vi "setROI.vi"(8 "error in (no error)":errorcluster, 10 "Coordinates":i32[](array[numeric]), 11 "ImageStreamViewer in":refnum<class "ImageStreamViewer.lvclass">) -> (0 "error out":errorcluster, 3 "ImageStreamViewer out":refnum<class "ImageStreamViewer.lvclass">)   [LabVIEW 2009, in "Views.lvlib" / "Camera.lvlib" / "ImageStreamViewer.lvclass"]
uses:
  ImageStreamViewer.lvclass
  ImageStreamViewer.lvclass/ImageStreamViewer.ctl
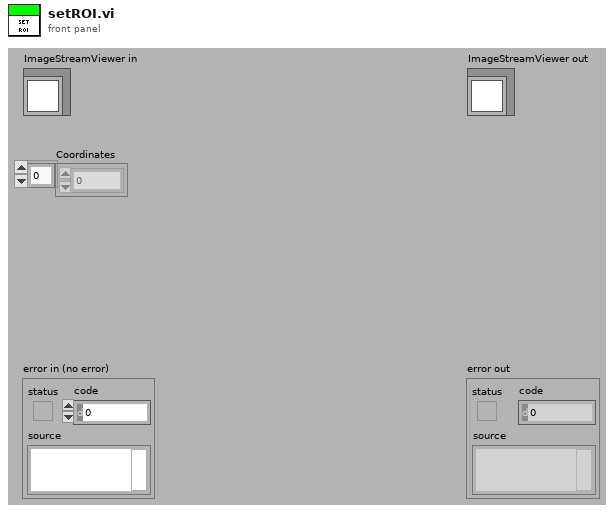
[diagram p1: front panel]
types:
  T1 = cluster{"Left":i32, "Top":i32, "Right":i32, "Bottom":i32}
  T2 = typedef "IMAQ Image.ctl" = refnum<image>
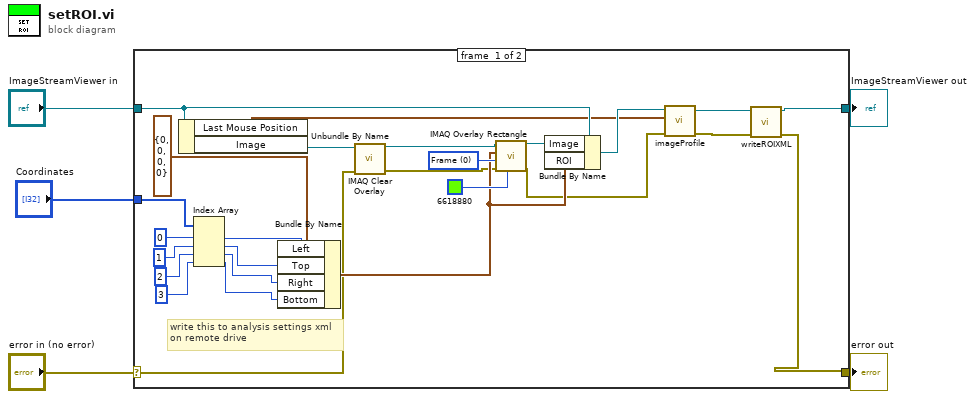
[diagram p0: block diagram]
diagram:
  n1 = case shown="No Error" "error in (no error)" {
    selector: "error in (no error)" -> [w14 w33]
    tunnel: [w7 w33] -> w4
    tunnel: [w6 w32] -> w2
    tunnel: "ImageStreamViewer in" -> [w23 w32]
    tunnel: "Coordinates" -> [w31 _]
    frame #0 {
      w26 = u32 0 items=["Frame", "Fill", "Highlight"] ("Drawing Mode (Frame)")
      # "write this to analysis settings xml\non remote drive"
      n2 = Unbundle By Name(w23) -> ("Last Mouse Position"=w10:cluster{"X":i32, "Y":i32}, "Image"=w15:T2)
      n3 = Index Array(array=w31, index #1=0, index #2=1, index #3=2, index #4=3) -> (element #1=w22:i32, element #2=w21:i32, element #3=w20:i32, element #4=w19:i32)
      n4 = Bundle By Name(cluster=T1 {"Left"=0, "Top"=0, "Right"=0, "Bottom"=0} ("Rectangle"), "Left"=w22, "Top"=w21, "Right"=w20, "Bottom"=w19) -> (w17:T1)
      n5 = call "IMAQ Clear Overlay"("error in (no error)"=w14, "Image"=w15) -> ("error out"=w13:errorcluster, "Image Out"=w16:T2)  [unwired: 8 in]
      n6 = call "IMAQ Overlay Rectangle"("Color"=u32 6618880, "error in (no error)"=w13, "Drawing Mode (Frame)"=w26, "Rectangle"=w17, "Image"=w16) -> ("error out"=w11:errorcluster, "Image Out"=w24:T2)  [unwired: 5 in]
      n7 = Bundle By Name(cluster=w23, "Image"=w24, "ROI"=w17) -> (w12:refnum<class "ImageStreamViewer.lvclass">)
      n8 = call "imageProfile.vi"("error in (no error)"=w11, "Point"=w10, "ImageStreamViewer in"=w12) -> ("error out"=w8:errorcluster, "ImageStreamViewer out"=w9:refnum<class "ImageStreamViewer.lvclass">)  [unwired: 7 in]
      n9 = call "writeROIXML.vi"("error in (no error)"=w8, "ImageStreamViewer in"=w9) -> ("error out"=w7:errorcluster, "ImageStreamViewer out"=w6:refnum<class "ImageStreamViewer.lvclass">)  [unwired: 8 in]
    }
    frame #1 {
    }
  }
  "error out" <- w4
  "ImageStreamViewer out" <- w2
